vi "TestControlVi_3.vi"() -> ()   [LabVIEW 2018]
panel:
  out "output cluster":cluster{"Sine with Uniform Noise":dynamicdata}
  out "Sine with Uniform Noise":dbl=0.05394995810837566
  in  "stop":bool
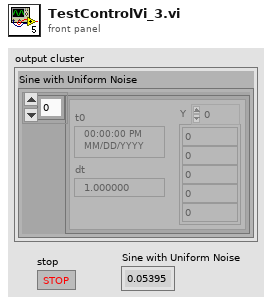
[diagram p1: front panel]
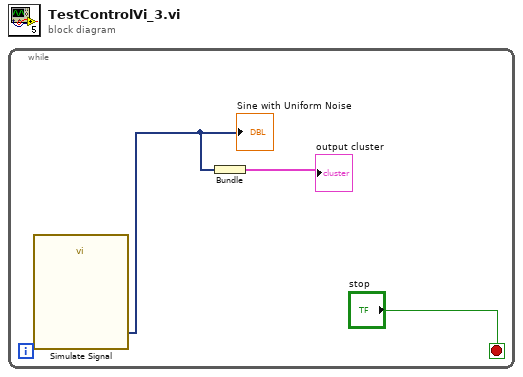
[diagram p0: block diagram]
diagram:
  n1 = while {
    stop <- "stop" stop-if-true
    n2 = call "Simulate Signal"() -> ("Sine with Uniform Noise"=w2:dynamicdata)  [unwired: 14 in, 1 out]
    "Sine with Uniform Noise" <- w2
    n3 = Bundle("Sine with Uniform Noise"=w2) -> (→"output cluster":cluster{"Sine with Uniform Noise":dynamicdata})  [unwired: 1 in]
  }
